vi "SerialMarvinMod.vi"(8 "error in (no error)":errorcluster, 9 "Clear Log":bool, 10 "write buffer":string="UA[3]\r\n", 11 "VISA resource name":refnum<visa-resource-name>="COM6") -> (0 "error out":errorcluster, 2 "read buffer":string)   [LabVIEW 2017]
uses:
  <vilib>/Instr/_visa.llb/VISA Configure Serial Port (Instr).vi
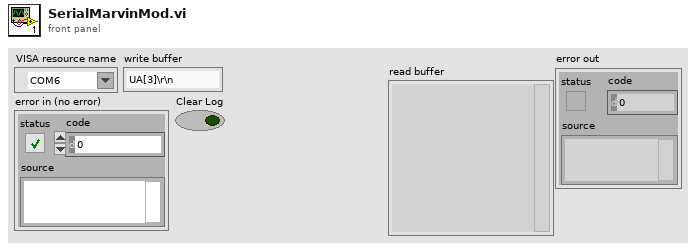
[diagram p1: front panel]
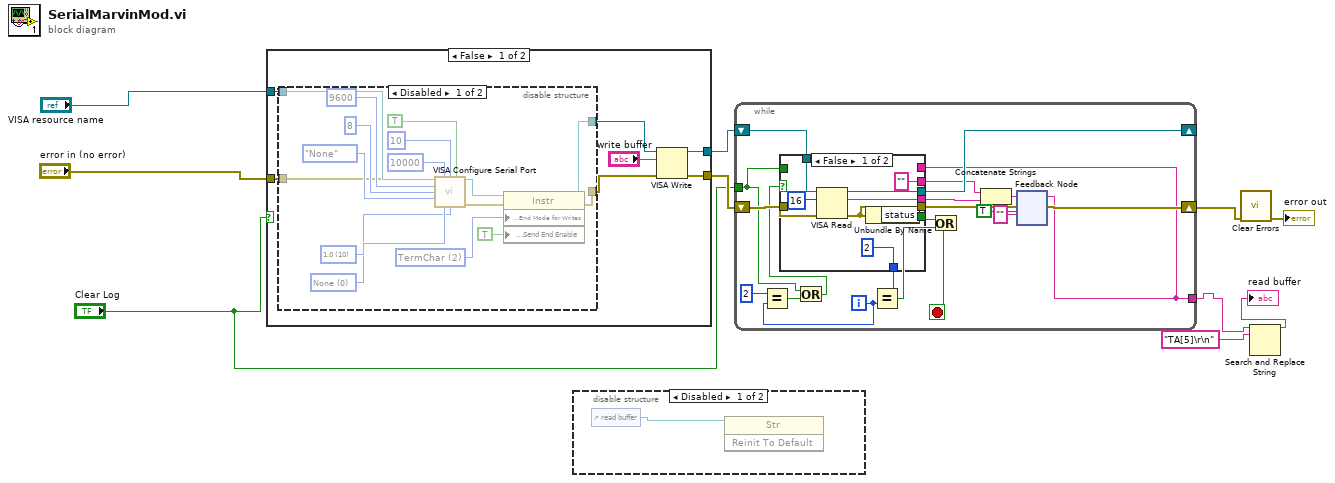
[diagram p0: block diagram]
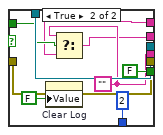
[diagram p5: hidden frame]
diagram:
  n1 = case shown="False" "Clear Log" {
    tunnel: "VISA resource name" -> [w17 w37]
    tunnel: "error in (no error)" -> [w16 w36]
    tunnel: [w13 w37] -> w6
    tunnel: [w12 w36] -> w5
    frame False {
      n2 = disable-structure shown="Disabled" {
        disable-tunnel: w17 -> [w33 w35]
        disable-tunnel: w16 -> [w27 w34]
        disable-tunnel: [w22 w35] -> w14
        disable-tunnel: [w21 w34] -> w15
        frame Disabled {
          w19 = u16 2 items=["None", "LastBit", "TermChar", "Break"] ("Serial Settings:Serial End Mode for Writes")
          w25 = u16 0 items=["None", "XON/XOFF", "RTS/CTS", "XON/XOFF & RTS/CTS", "DTR/DSR", "XON/XOFF & DTR/DSR"] ("flow control (0:none)")
          w26 = u16 10 items=["1.0"=10, "1.5"=15, "2.0"=20] ("stop bits (10: 1 bit)")
          n3 = call-poly "VISA Configure Serial Port"("VISA resource name"=w33, "timeout (10sec)"=u32 10000, "termination char\n(0xA = '\\n' = LF)"=u8 10 ("termination char\n(0xA = '\\n' = LF)"), "Enable Termination\nChar (T)"=TRUE ("Enable Termination\nChar (T)"), "baud rate (9600)"=u32 9600, "data bits (8)"=u16 8, "parity (0:none)"=enum16{"None", "Odd", "Even", "Mark", "Space"}."None", "error in (no error)"=w27, "stop bits (10: 1 bit)"=w26, "flow control (0:none)"=w25) -> ("VISA resource name out"=w23:refnum<visa-resource-name>, "error out"=w24:errorcluster)  [unwired: 4 in]
          n4 = property class="Instr"(reference=w23, error in=w24, "Serial Settings:End Mode for Writes"=w19, "Message Based Settings:Send End Enable"=TRUE) -> (reference out=w22:refnum<visa-resource-name>, error out=w21:errorcluster)
        }
        frame Enabled {
        }
      }
      n5 = VISA Write(VISA resource name=w14, write buffer="write buffer", error in (no error)=w15) -> (VISA resource name out=w13:refnum<visa-resource-name>, error out=w12:errorcluster)  [unwired: 1 out]
    }
    frame True {
    }
  }
  n6 = disable-structure shown="Disabled" {
    frame Disabled {
      n7 = control-ref of="read buffer"() -> (w38:refnum<vi>)
      n8 = invoke class="Str" method="Reinit To Default"(reference=w38) -> ()  [unwired: 2 in, 3 out]
    }
    frame Enabled {
    }
  }
  n9 = while {
    shift-right: [w57] -> _
    shift-left: w6 -> [w51]
    shift-right: [w55] -> w9
    shift-left: w5 -> [w50]
    tunnel: [w48] -> w3
    tunnel: "Clear Log" -> [w41]
    i -> [w45]
    stop <- w53 stop-if-true
    n10 = Equal?(x=2, y=w45) -> (x = y?=w43:bool)
    n11 = Or(x=w41, y=w43) -> (x .or. y?=w42:bool)
    n12 = feedback #1("") -> (w48:string)
    n13 = case shown="False" w42 {
      tunnel: [w66 w75] -> w57
      tunnel: [w65 w69] -> w56
      tunnel: [w63 w74] -> w55
      tunnel: [w62 FALSE ("status")] -> w52
      tunnel: w51 -> [w61 w75]
      tunnel: w50 -> [w60 w74]
      tunnel: w48 -> [_ w68]
      tunnel: ["" w67] -> w47
      tunnel: [2 ("x") 2 ("x")] -> w46
      tunnel: w41 -> [_ w70]
      frame False {
        n14 = VISA Read(VISA resource name=w61, byte count=u32 16, error in (no error)=w60) -> (VISA resource name out=w66:refnum<visa-resource-name>, read buffer=w65:string, error out=w63:errorcluster)  [unwired: 1 out]
        n15 = Unbundle By Name(w63) -> ("status"=w62:bool)
      }
      frame True {
        w69 = ""
        n16 = property on="Clear Log" class="Bool (strict)"("Value"=FALSE ("Clear Log")) -> ()  [unwired: 2 in, 2 out]
        n17 = Select(t=w69, s=w70, f=w68) -> (s? t:f=w67:string)
      }
    }
    n18 = Equal?(x=w46, y=w45) -> (x = y?=w54:bool)
    n19 = Or(x=w52, y=w54) -> (x .or. y?=w53:bool)
    n20 = Concatenate Strings(w47, w56) -> (w49:string)
    n21 = feedback-in #1(w49, TRUE) -> ()
  }
  n22 = call <vilib>:"Clear Errors.vi"("error in (no error)"=w9) -> ("error out"=→"error out":errorcluster)  [unwired: 5 in, 1 out]
  n23 = Search and Replace String(input string=w3, search string="TA[5]\r\n" ("substring (\"\")")) -> (result string=→"read buffer":string)  [unwired: 6 in, 3 out]
